vi "CLD 12 Sequencer State Machine.vi"() -> ()   [LabVIEW 2020]
doc: "CLD 12 exercise"
panel:
  out "Error Out":errorcluster
  in  "Error In":errorcluster
  out "Current Time Target":dbl
  in  "Stop Button":bool
  out "Time Elapsed":dbl
  out "Switch 3":bool
  out "Switch 2":bool
  out "Switch 1":bool
  in  "Start":bool
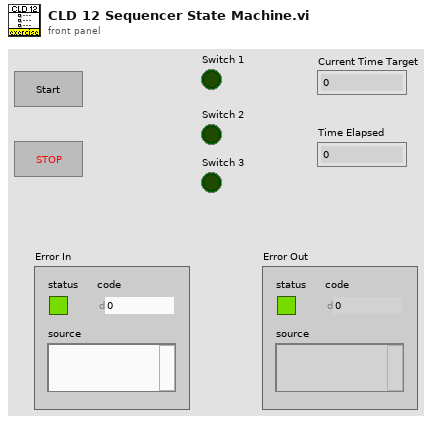
[diagram p1: front panel]
types:
  T1 = typedef "CLD 8 Data Cluster.ctl" = cluster{"Command":string, "Time":string, "Indicator1":bool, "Indicator2":bool, "Indicator3":bool}
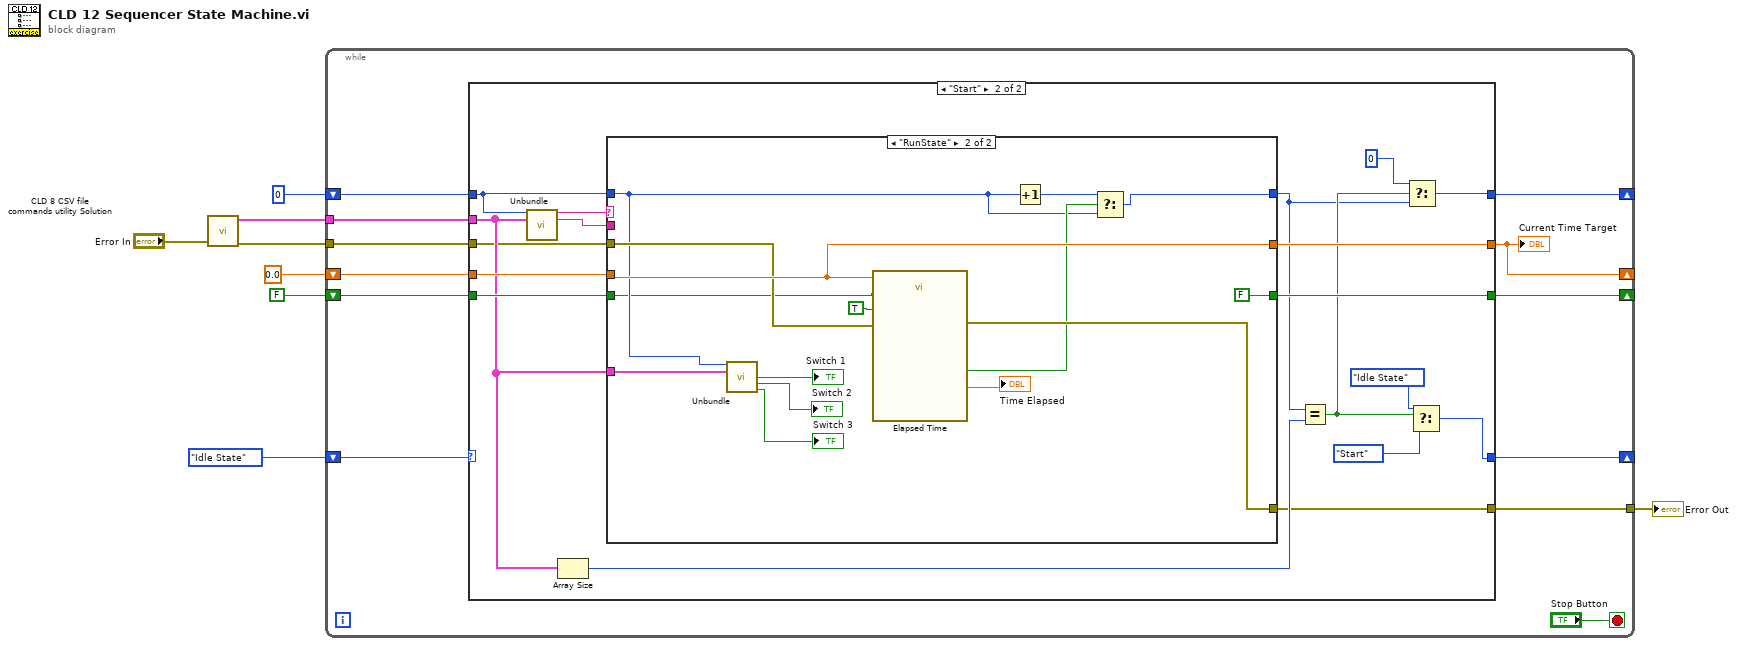
[diagram p0: block diagram]
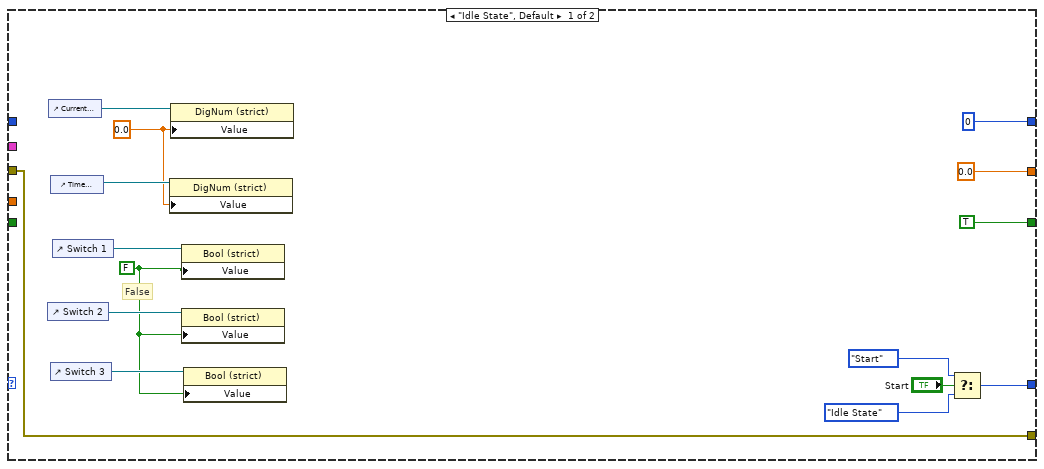
[diagram p2: hidden frame]
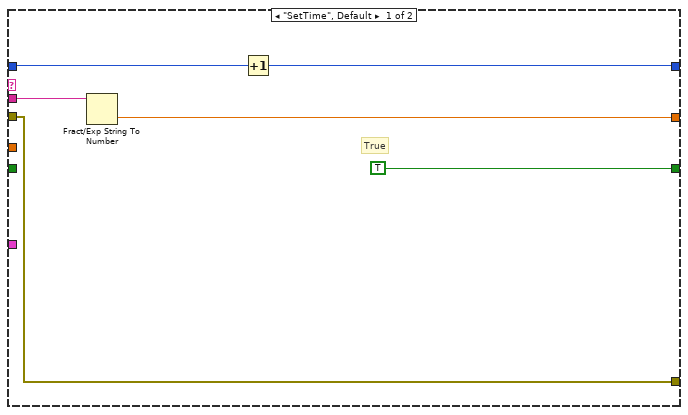
[diagram p3: hidden frame]
diagram:
  n1 = call "CLD 8 CSV file commands utility Solution.vi"("Error In"="Error In") -> ("Error Out"=w3:errorcluster, "Commands Out Array"=w7:T1[])  [unwired: 9 in]
  n2 = while {
    shift-right: [w18] -> _
    shift-left: enum16{"Idle State", "Start"}."Idle State" -> [w19]
    tunnel: w7 -> [w17]
    shift-right: [w15] -> _
    shift-left: 0 ("index") -> [w16]
    shift-right: [w11] -> _
    shift-left: 0.0 -> [w14]
    shift-right: [w12] -> _
    shift-left: FALSE ("Reset") -> [w13]
    tunnel: w3 -> [w10]
    tunnel: [w9] -> w1
    stop <- "Stop Button" stop-if-true
    n3 = case shown="\"Start\"" w19 {
      tunnel: [w22 w42] -> w18
      tunnel: w17 -> [_ w46]
      tunnel: w16 -> [_ w52]
      tunnel: [0 ("t") w38] -> w15
      tunnel: w14 -> [_ w51]
      tunnel: [0.0 w49] -> w11
      tunnel: w13 -> [_ w48]
      tunnel: [TRUE ("Switch 1") w47] -> w12
      tunnel: w10 -> [w21 w37]
      tunnel: [w21 w36] -> w9
      frame "Idle State", Default {
        w29 = FALSE ("Value")
        w33 = 0.0 ("Value")
        # "False"
        n4 = control-ref of="Switch 2"() -> (w31:refnum<vi>)
        n5 = control-ref of="Current Time Target"() -> (w35:refnum<vi>)
        n6 = control-ref of="Time Elapsed"() -> (w34:refnum<vi>)
        n7 = control-ref of="Switch 3"() -> (w30:refnum<vi>)
        n8 = control-ref of="Switch 1"() -> (w32:refnum<vi>)
        n9 = property class="DigNum (strict)"(reference=w34, "Value"=w33) -> ()  [unwired: 1 in, 2 out]
        n10 = property class="DigNum (strict)"(reference=w35, "Value"=w33) -> ()  [unwired: 1 in, 2 out]
        n11 = property class="Bool (strict)"(reference=w32, "Value"=w29) -> ()  [unwired: 1 in, 2 out]
        n12 = property class="Bool (strict)"(reference=w31, "Value"=w29) -> ()  [unwired: 1 in, 2 out]
        n13 = property class="Bool (strict)"(reference=w30, "Value"=w29) -> ()  [unwired: 1 in, 2 out]
        n14 = Select(t=enum16{"Idle State", "Start"}."Start", s="Start", f=enum16{"Idle State", "Start"}."Idle State") -> (s? t:f=w22:enum16{"Idle State", "Start"})
      }
      frame "Start" {
        n15 = call "Unbundle.vi"("index"=w52, "Commands Out Array"=w46) -> ("Command"=w53:string, "Time"=w50:string)  [unwired: 9 in, 3 out]
        n16 = Array Size(array=w46) -> (size(s)=w45:i32)
        n17 = case shown="\"RunState\"" w53 {
          tunnel: w51 -> [_ w72]
          tunnel: w52 -> [w56 w63]
          tunnel: [w55 w60] -> w40
          tunnel: w50 -> [w59 _]
          tunnel: [w58 w72] -> w49
          tunnel: w48 -> [_ w62]
          tunnel: [TRUE ("Switch 1") FALSE ("Switch 1")] -> w47
          tunnel: w46 -> [_ w73]
          tunnel: w37 -> [w54 w71]
          tunnel: [w54 w70] -> w36
          frame "SetTime", Default {
            # "True"
            n18 = Fract/Exp String To Number(string=w59) -> (number=w58:dbl)  [unwired: 3 in, 1 out]
            n19 = Increment(x=w56) -> (x+1=w55:i32)
          }
          frame "RunState" {
            n20 = call "Unbundle.vi"("index"=w63, "Commands Out Array"=w73) -> ("Indicator1"=→"Switch 1":bool, "Indicator2"=→"Switch 2":bool, "Indicator3"=→"Switch 3":bool)  [unwired: 9 in, 2 out]
            n21 = call "Elapsed Time"("Time Target (s)"=w72, "Reset"=w62, "Auto Reset"=TRUE, "error in (no error)"=w71) -> ("Elapsed Time (s)"=→"Time Elapsed":dbl, "Time has Elapsed"=w64:bool, "error out"=w70:errorcluster)  [unwired: 8 in, 5 out]
            n22 = Increment(x=w63) -> (x+1=w65:i32)
            n23 = Select(t=w65, s=w64, f=w63) -> (s? t:f=w60:i32)
          }
        }
        n24 = Equal?(x=w40, y=w45) -> (x = y?=w41:bool)
        n25 = Select(t=0, s=w41, f=w40) -> (s? t:f=w38:i32)
        n26 = Select(t=enum16{"Idle State", "Start"}."Idle State", s=w41, f=enum16{"Idle State", "Start"}."Start") -> (s? t:f=w42:enum16{"Idle State", "Start"})
      }
    }
    "Current Time Target" <- w11
  }
  "Error Out" <- w1
